vi "Calibrate Helmet.vi"(8 "Error In":errorcluster) -> (0 "Error Out":errorcluster)   [LabVIEW 2020]
panel:
  in  "stop (F)":bool caption="Stop (F)"
  out "Pressure":dbl[](array[numeric])
  out "Flow":dbl[](array[numeric])
  out "XY Graph":cluster{"Y":dbl[], "Y":dbl[]}[](graph)
  out "Offset":dbl
  out "Gain":dbl
  in  "Flow":dbl
  out "Pressure (V)":dbl format="%.4f"
  out "Chart":dynamicdata(graph)
  in  "Add":bool
  # "Flow"
  # "Pressure"
  # "Calculated Gain"
  # "Offset"
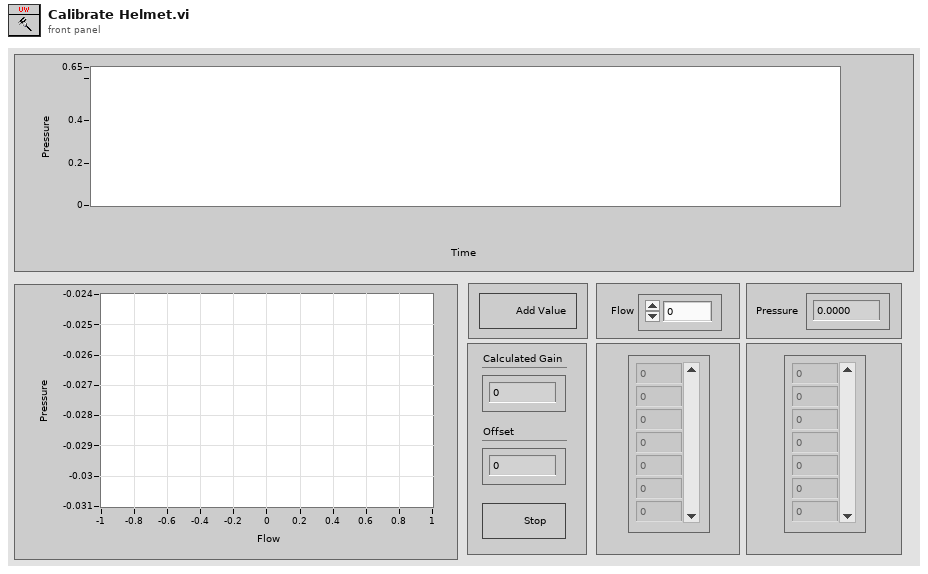
[diagram p1: front panel]
types:
  T1 = enum16{"open", "replace", "create", "open or create", "replace or create", "replace or create with confirmation"}
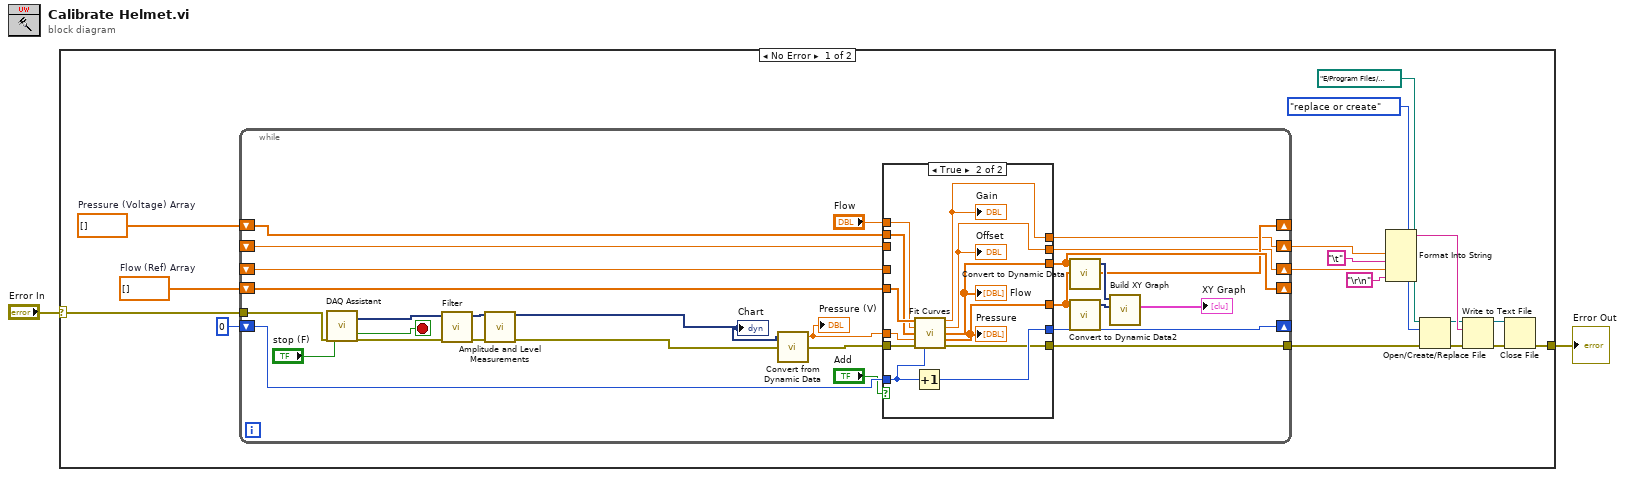
[diagram p0: block diagram]
diagram:
  n1 = case shown="No Error" "Error In" {
    selector: "Error In" -> [w3 w64]
    tunnel: [w11 w64] -> w1
    frame No Error {
      w17 = dbl[] []  # Pressure (Voltage) Array
      w19 = dbl[] []  # Flow (Ref) Array
      n2 = while {
        tunnel: w3 -> [w45]
        shift-right: [w38] -> _
        shift-left: w19 -> [w33]
        shift-right: [w37] -> _
        shift-left: w17 -> [w32]
        shift-right: [w35] -> _
        shift-left: 0 ("index") -> [w36]
        tunnel: [w31] -> w10
        shift-right: [w30] -> w5
        shift-left: _ -> [w28]
        shift-right: [w29] -> w4
        shift-left: _ -> [w27]
        stop <- w43 stop-if-true
        n3 = call "DAQ Assistant"("error in"=w45, "stop (F)"="stop (F)") -> ("data"=w25:dynamicdata, "stopped"=w43:bool, "error out"=w26:errorcluster)  [unwired: 14 in, 1 out]
        n4 = call "Filter"("error in (no error)"=w26, "Signal"=w25) -> ("error out"=w24:errorcluster, "Filtered Signal"=w23:dynamicdata)  [unwired: 8 in]
        n5 = call "Amplitude and Level Measurements"("Signals"=w23, "error in (no error)"=w24) -> ("Mean (DC)"=w21:dynamicdata, "error out"=w20:errorcluster)  [unwired: 12 in]
        "Chart" <- w21
        n6 = call "Convert from Dynamic Data"("Dynamic Data Type"=w21) -> ("Scalar"=w22:dbl)  [unwired: 3 in]
        "Pressure (V)" <- w22
        n7 = case shown="True" "Add" {
          tunnel: "Flow" -> [_ w58]
          tunnel: [w51 w55] -> w38
          tunnel: [w50 w54] -> w37
          tunnel: w32 -> [w50 w57]
          tunnel: w33 -> [w51 w59]
          tunnel: w36 -> [w49 w62]
          tunnel: [w49 w63] -> w35
          tunnel: w20 -> [w48 w61]
          tunnel: [w48 w60] -> w31
          tunnel: w22 -> [_ w56]
          tunnel: [w47 w53] -> w30
          tunnel: [w46 w52] -> w29
          tunnel: w28 -> [w47 _]
          tunnel: w27 -> [w46 _]
          frame False {
          }
          frame True {
            n8 = Increment(x=w62) -> (x+1=w63:i32)
            n9 = call "Fit Curves.vi"("Reference (Array)"=w59, "Reference (Value)"=w58, "Voltage (Array)"=w57, "Voltage (Value)"=w56, "Error In"=w61, "index"=w62) -> ("Slope"=w53:dbl, "Intercept"=w52:dbl, "Reference Out"=w55:dbl[], "Voltage Out"=w54:dbl[], "Error Out"=w60:errorcluster)  [unwired: 5 in]
            "Gain" <- w53
            "Offset" <- w52
            "Flow" <- w55
            "Pressure" <- w54
          }
        }
        n10 = call "Convert to Dynamic Data"("Array"=w38) -> ("Dynamic Data Type"=w40:dynamicdata)  [unwired: 3 in]
        n11 = call "Convert to Dynamic Data2"("Array"=w37) -> ("Dynamic Data Type"=w39:dynamicdata)  [unwired: 3 in]
        n12 = call "Build XY Graph"("Y Input"=w39, "X Input"=w40) -> ("XY Graph"=→"XY Graph":cluster{"Y":dbl[], "Y":dbl[]}[])  [unwired: 8 in, 1 out]
      }
      n13 = Format Into String(w5, "\t", w4, "\r\n") -> (resulting string=w14:string)  [unwired: 3 in, 1 out]
      n14 = Open/Create/Replace File(file path (use dialog)=path "E:/Program Files/Master Aero Program/Calibration .txt files/SH Cali.txt", error in=w10, operation (0:open)=T1."replace or create") -> (refnum out=w12:refnum<file>, error out=w15:errorcluster)  [unwired: 3 in, 1 out]
      n15 = Write to Text File(file (use dialog)=w12, text=w14, error in=w15) -> (refnum out=w13:refnum<file>, error out=w16:errorcluster)  [unwired: 1 in, 1 out]
      n16 = Close File(refnum=w13, error in=w16) -> (error out=w11:errorcluster)  [unwired: 1 out]
    }
    frame Error {
    }
  }
  "Error Out" <- w1
